vi "GetControls.vi"(6 "error in":errorcluster, 9 "Tab in":refnum<class "Tab.lvclass">) -> (0 "error out":errorcluster, 3 "Tab out":refnum<class "Tab.lvclass">, 4 "Controls":cluster{"controls":i32[], "decorations":i32[]}[](array[cluster]))   [LabVIEW 2014, in "Raspberry Pi Compatible Compiler for LabVIEW.lvlib" / "Tab.lvclass"]
uses:
  Tab.lvclass
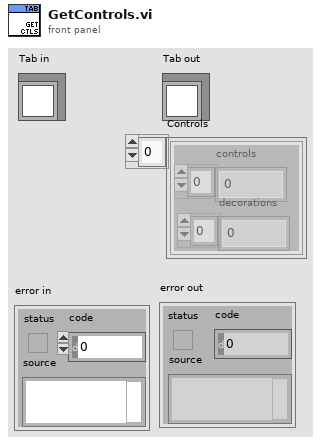
[diagram p1: front panel]
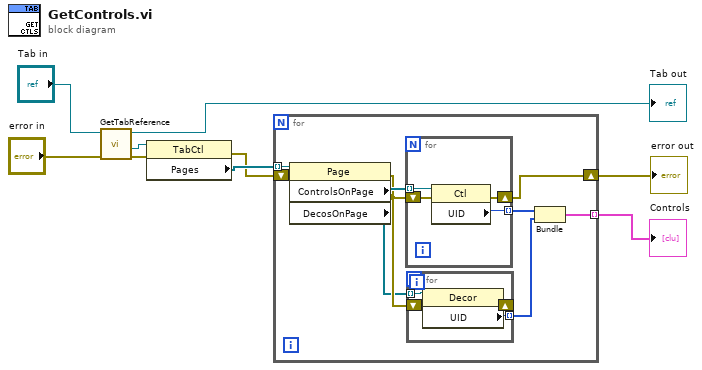
[diagram p0: block diagram]
diagram:
  n1 = call "GetTabReference.vi"("error in"="error in", "Tab in"="Tab in") -> ("error out"=w6:errorcluster, "tab reference"=w7:refnum<vi>, "Tab out"=→"Tab out":refnum<class "Tab.lvclass">)  [unwired: 7 in]
  n2 = property class="TabCtl"(reference=w7, error in=w6) -> (error out=w4:errorcluster, "Pages"=w5:refnum<vi>[])  [unwired: 1 out]
  n3 = for {
    tunnel: w5 -> [w17] mode=indexing
    shift-right: [w14] -> w2
    shift-left: w4 -> [w18]
    tunnel: [w13] -> w1 mode=indexing
    n4 = property class="Page"(reference=w17, error in=w18) -> (error out=w12:errorcluster, "ControlsOnPage"=w16:refnum<vi>[], "DecosOnPage"=w11:refnum<vi>[])  [unwired: 1 out]
    n5 = for {
      tunnel: w16 -> [w25] mode=indexing
      shift-right: [w24] -> w14
      shift-left: w12 -> [w26]
      tunnel: [w23] -> w15 mode=indexing
      n6 = property class="Ctl"(reference=w25, error in=w26) -> (error out=w24:errorcluster, "UID"=w23:i32)  [unwired: 1 out]
    }
    n7 = for {
      tunnel: w11 -> [w21] mode=indexing
      shift-right: [w20] -> _
      shift-left: w12 -> [w22]
      tunnel: [w19] -> w10 mode=indexing
      n8 = property class="Decor"(reference=w21, error in=w22) -> (error out=w20:errorcluster, "UID"=w19:i32)  [unwired: 1 out]
    }
    n9 = Bundle(w15, w10) -> (w13:cluster{i32[], i32[]})  [unwired: 1 in]
  }
  "error out" <- w2
  "Controls" <- w1
